vi "Get Obj Data.vi"(0 "reference in":refnum<class "RPC.lvclass">, 5 "error in (no error)":errorcluster) -> (14 "reference out":refnum<class "RPC.lvclass">, 17 "Time Data":refnum<class "GSwFormDSP.lvclass">, 19 "error out":errorcluster)   [LabVIEW 2022 SP3, in "RPC.lvclass"]
uses:
  RPC.lvclass
  API/GSwFormDSP_class/GSwFormDSP.lvclass
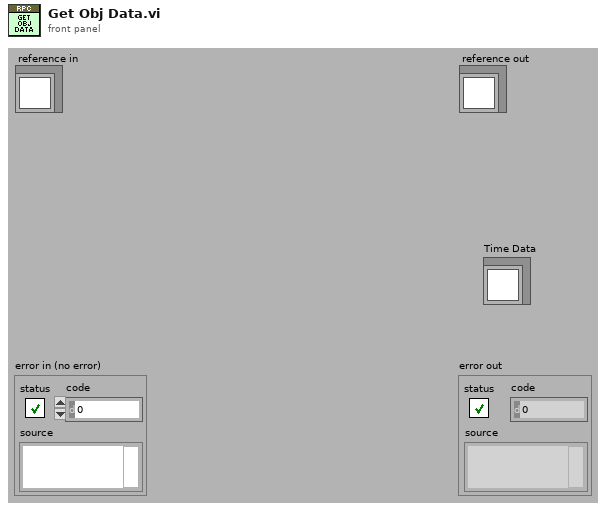
[diagram p1: front panel]
types:
  T1 = typedef "RPC.lvclass/ObjectAttributes.ctl" = cluster{"File Refnum":refnum<file>, "File total size":i32, "Offset from start of file":i32, "Time Type":enum16{"Response", "Drive"}, "Full Scale":dbl[unit], "New Time Data Obj?":bool, "Header":cluster{"Num Header":i32, "Num Parameter":i32, "Nb Channels":i32, "dT":dbl, "Number of Groups":i32, "Group size":i32, "Units":string[], "Names":string[], "Sensitivity":dbl[], "Complete header":string[]}, "Time Data":refnum<class "GSwFormDSP.lvclass">}
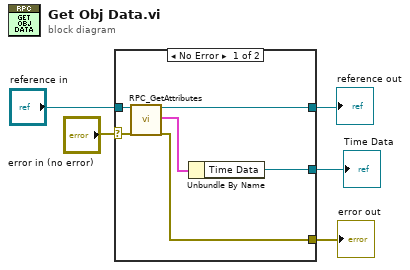
[diagram p0: block diagram]
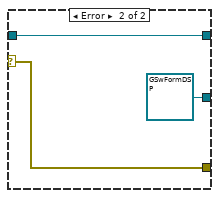
[diagram p2: hidden frame]
diagram:
  n1 = case shown="No Error" "error in (no error)" {
    selector: "error in (no error)" -> [w11 w14]
    tunnel: [w10 w14] -> w4
    tunnel: [w9 w13] -> w2
    tunnel: "reference in" -> [w7 w13]
    tunnel: [w6 refnum<class "GSwFormDSP.lvclass"> refnum ("Time Data")] -> w1
    frame No Error {
      n2 = call "RPC_GetAttributes.vi"("reference in"=w7, "error in (no error)"=w11) -> ("reference out"=w9:refnum<class "RPC.lvclass">, "attributes"=w8:T1, "error out"=w10:errorcluster)  [unwired: 14 in, 1 out]
      n3 = Unbundle By Name(w8) -> ("Time Data"=w6:refnum<class "GSwFormDSP.lvclass">)
    }
    frame Error {
    }
  }
  "error out" <- w4
  "reference out" <- w2
  "Time Data" <- w1
